vi "EnumerateSerialPortsph.vi"() -> (2 "names":string[](array[string]))   [LabVIEW 2010]
panel:
  in  "application reference (local)":refnum<vi>
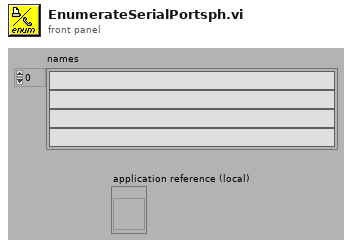
[diagram p1: front panel]
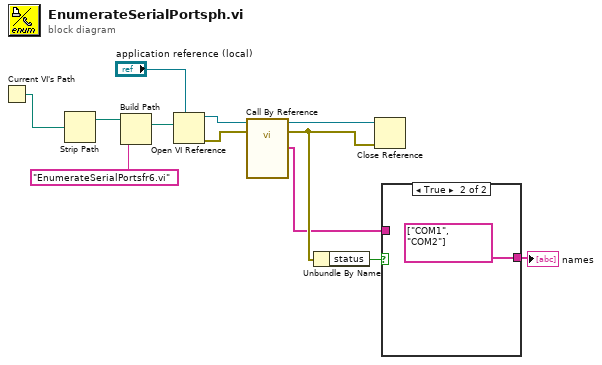
[diagram p0: block diagram]
diagram:
  n1 = Current VI's Path() -> (path=w4:path)
  n2 = Strip Path(path=w4) -> (stripped path=w3:path)  [unwired: 1 out]
  n3 = Build Path(base path=w3, name or relative path="EnumerateSerialPortsfr6.vi") -> (appended path=w1:path)
  n4 = Open VI Reference(type specifier VI Refnum (for type only)="application reference (local)", vi path=w1) -> (vi reference=w11:refnum<vi>, error out=w10:errorcluster)  [unwired: 4 in]
  n5 = call-by-ref "?"(reference=w11, error in=w10) -> (reference out=w9:refnum<vi>, error out=w8:errorcluster, "names"=w5:string[])  [unwired: 2 out]
  n6 = Unbundle By Name(w8) -> ("status"=w7:bool)
  n7 = Close Reference(reference=w9, error in (no error)=w8) -> ()  [unwired: 1 out]
  n8 = case shown="True" w7 {
    tunnel: [w13 string[] ["COM1", "COM2"] ("names")] -> w6
    tunnel: w5 -> [w13 _]
    frame False {
    }
    frame True {
    }
  }
  "names" <- w6
